vi "MeanPolyFitNaN.vi"(11 "Data":dbl[][](array[numeric])) -> (2 "Polynomial Coefficients":dbl[](array[numeric]), 3 "Best Polynomial Fit":dbl[](array[numeric]))   [LabVIEW 2014, in "Head Impulse Fit.lvclass"]
uses:
  Head Impulse Fit.lvclass
  <vilib>/Analysis/6fits.llb/General Linear Fit Algorithm.ctl
  <vilib>/Analysis/1siggen.llb/Ramp Pattern by Samples.vi
  <vilib>/Analysis/polynomials.llb/1D Polynomial Evaluation (DBL).vi
  <vilib>/Analysis/NI_AALBase.lvlib
  <vilib>/Analysis/NI_AALPro.lvlib
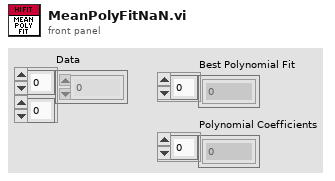
[diagram p1: front panel]
types:
  T1 = typedef "NI_AALPro.lvlib/General Linear Fit Algorithm.ctl" = u16
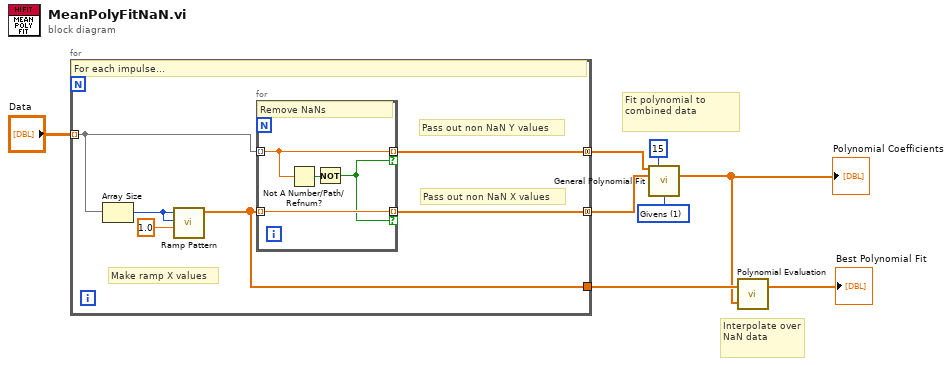
[diagram p0: block diagram]
diagram:
  w7 = T1 1 items=["SVD", "Givens", "Givens2", "Householder", "LU Decomposition", "Cholesky", "SVD for Rank Deficient H"] ("algorithm")
  # "Interpolate over NaN data"
  # "Fit polynomial to combined data"
  n1 = for {
    tunnel: "Data" -> [w12] mode=indexing
    tunnel: [w11] -> w4 mode=concatenating
    tunnel: [w10] -> w5 mode=concatenating
    tunnel: [w9] -> w3
    # "Pass out non NaN X values"
    # "Pass out non NaN Y values"
    # "Make ramp X values"
    # "For each impulse..."
    n2 = Array Size(array=w12) -> (size(s)=w13:i32)
    n3 = call-poly <vilib>:"Ramp Pattern.vi"("start"=1.0, "end"=w13, "samples"=w13) -> ("Ramp Pattern"=w9:dbl[])  [unwired: 7 in, 1 out]
    n4 = for {
      tunnel: w12 -> [w18] mode=indexing
      tunnel: w9 -> [w17] mode=indexing
      tunnel: [w18] -> w10 mode=indexing if=w15
      tunnel: [w17] -> w11 mode=indexing if=w15
      # "Remove NaNs"
      n5 = Not A Number/Path/Refnum?(number/path/refnum=w18) -> (NaN/Path/Refnum?=w16:bool)
      n6 = Not(x=w16) -> (.not. x?=w15:bool)
    }
  }
  n7 = call <vilib>:"General Polynomial Fit.vi"("Y"=w5, "polynomial order"=15, "X"=w4, "algorithm"=w7) -> ("Polynomial Coefficients"=w2:dbl[])  [unwired: 8 in, 3 out]
  "Polynomial Coefficients" <- w2
  n8 = call-poly <vilib>:"Polynomial Evaluation.vi"("P(x)"=w2, "A"=w3) -> ("P(A)"=→"Best Polynomial Fit":dbl[])  [unwired: 1 out]
